vi "GCMPlugin_IsSupportingItem.vi"(8 "error in (no error)":errorcluster, 9 "VI Reference":refnum<vi>, 10 "ProjectItem Refnum":refnum<vi>, 11 "TemplatePlugin in":refnum<class "GCMSettingsScreen.lvclass">) -> (0 "error out":errorcluster, 2 "IsSupportingItem":bool, 3 "TemplatePlugin out":refnum<class "GCMSettingsScreen.lvclass">)   [LabVIEW 2014, in "GCMSettingsScreen.lvlib" / "GCMSettingsScreen.lvclass"]
uses:
  GCMSettingsScreen.lvclass
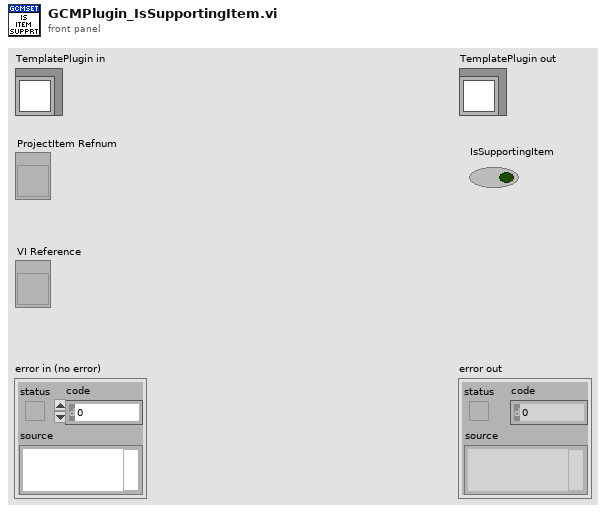
[diagram p1: front panel]
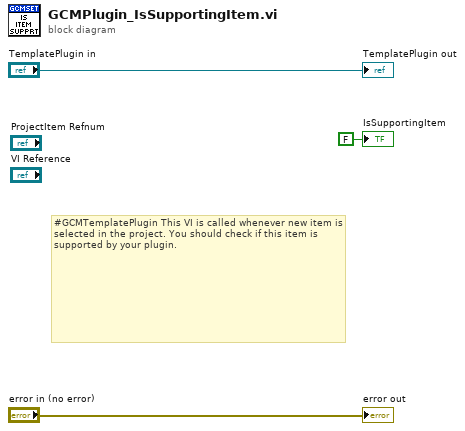
[diagram p0: block diagram]
diagram:
  # "#GCMTemplatePlugin This VI is called whenever new item is selected in the project. You should check if this item is supported by your plugin."
  "error out" <- "error in (no error)"
  "TemplatePlugin out" <- "TemplatePlugin in"
  "IsSupportingItem" <- FALSE ("IsSupportingItem")
